vi "Initial Path Plot Sub_VI.vi"(8 "error in (no error)":errorcluster, 10 "Motion Inputs":T3) -> (0 "error out":errorcluster, 1 "Accel Array":dbl[](graph), 2 "Velocity Array":dbl[](graph), 3 "Displacement Array":dbl[](graph), 4 "V max (mm/s)":dbl, 5 "Motion Points":T1, 6 "Dist max (mm)":dbl, 7 "Motion Outputs":T2)   [LabVIEW 2017]
panel:
  out "Waveform Chart":T1(graph)
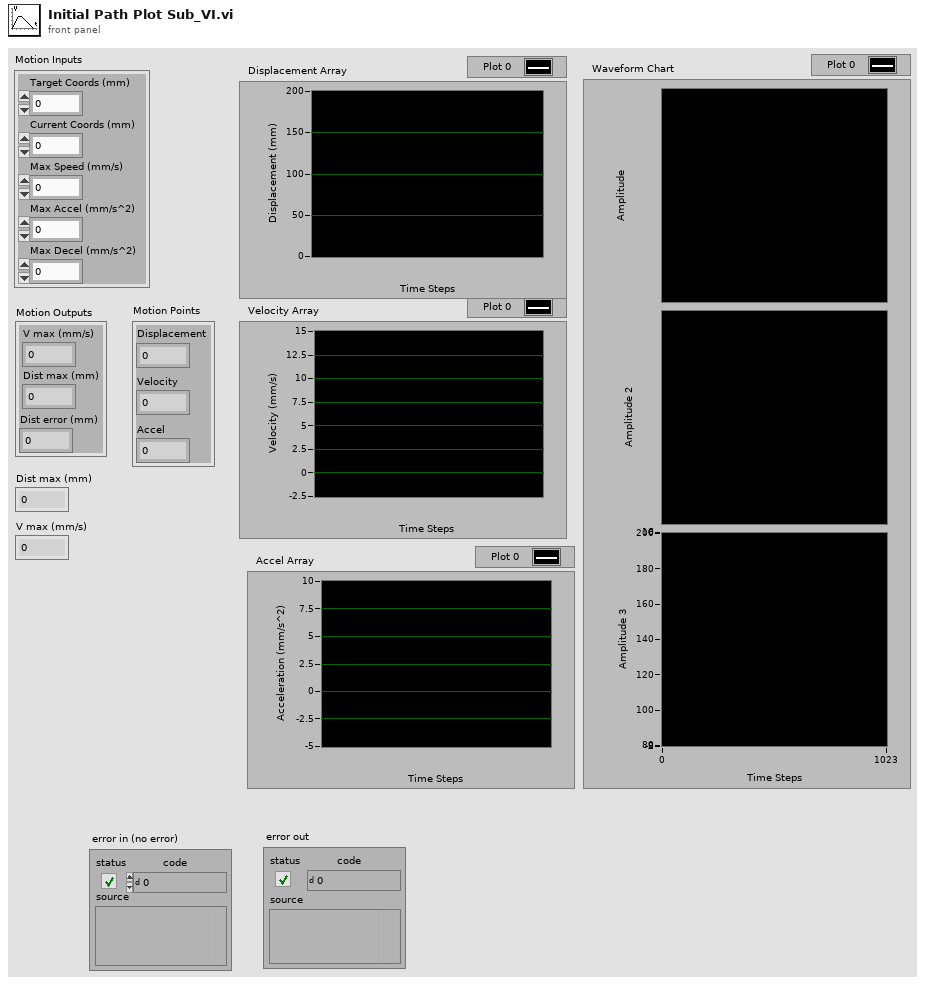
[diagram p1: front panel]
types:
  T1 = cluster{"Accel":dbl, "Velocity":dbl, "Displacement":dbl}
  T2 = cluster{"V max (mm/s)":dbl, "Dist max (mm)":dbl, "Dist error (mm)":dbl}
  T3 = cluster{"Target Coords (mm)":dbl, "Current Coords (mm)":dbl, "Max Speed (mm/s)":dbl, "Max Accel (mm/s^2)":dbl, "Max Decel (mm/s^2)":dbl}
  T4 = cluster{" Distance target (mm)":dbl, "Max Accel (mm/s^2)":dbl, "Max Decel (mm/s^2)":dbl, "Velocity Limit (mm/s) ":dbl, "Time step (s)":dbl}
  T5 = cluster{"Cruising Speed (mm/s)":dbl, "Crusing Time (s)":dbl, "Decel Time (s)":dbl, "Accel Time (s)":dbl, "Total Time (s)":dbl, "Accel Distance (mm)":dbl, "Decel Distance (mm)":dbl, "Crusing Distance (mm)":dbl}
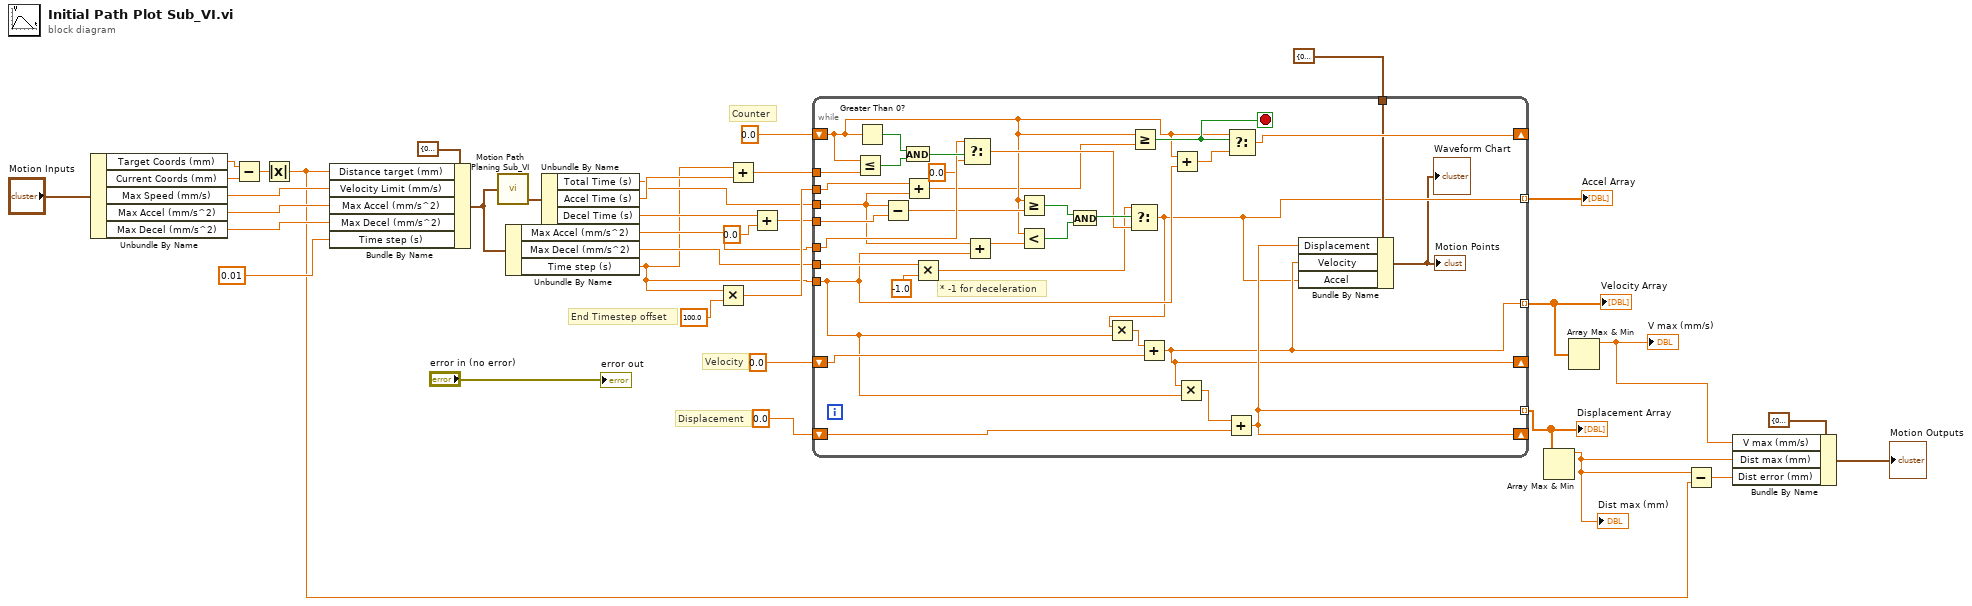
[diagram p0: block diagram]
diagram:
  # "End Timestep offset"
  # "Displacement"
  # "Velocity"
  # "Counter"
  n1 = Unbundle By Name("Motion Inputs") -> ("Target Coords (mm)"=w34:dbl, "Current Coords (mm)"=w35:dbl, "Max Speed (mm/s)"=w32:dbl, "Max Accel (mm/s^2)"=w31:dbl, "Max Decel (mm/s^2)"=w30:dbl)
  n2 = Subtract(x=w34, y=w35) -> (x-y=w21:dbl)
  n3 = Absolute Value(x=w21) -> (abs(x)=w24:dbl)
  n4 = Bundle By Name(cluster=T4 {" Distance target (mm)"=0.0, "Max Accel (mm/s^2)"=0.0, "Max Decel (mm/s^2)"=0.0, "Velocity Limit (mm/s) "=0.0, "Time step (s)"=0.0} ("Motion Planning Inputs"), "Distance target (mm)"=w24, "Velocity Limit (mm/s)"=w32, "Max Accel (mm/s^2)"=w31, "Max Decel (mm/s^2)"=w30, "Time step (s)"=0.01) -> (w28:T4)
  n5 = call "Motion Path Planing Sub_VI.vi"("Motion Planning Inputs"=w28) -> ("Motion Planning Outputs"=w26:T5)  [unwired: 4 in, 2 out]
  n6 = Unbundle By Name(w28) -> ("Max Accel (mm/s^2)"=w3:dbl, "Max Decel (mm/s^2)"=w2:dbl, "Time step (s)"=w1:dbl)
  n7 = Unbundle By Name(w26) -> ("Total Time (s)"=w5:dbl, "Accel Time (s)"=w6:dbl, "Decel Time (s)"=w4:dbl)
  n8 = Multiply(x=w1, y=100.0) -> (x*y=w19:dbl)
  n9 = Add(x=w1, y=w6) -> (x+y=w15:dbl)
  n10 = Add(x=w4, y=0.0) -> (x+y=w16:dbl)
  n11 = while {
    shift-right: [w47] -> _
    shift-left: 0.0 -> [w46]
    tunnel: w15 -> [w69]
    tunnel: w3 -> [w65]
    tunnel: w5 -> [w57]
    tunnel: w16 -> [w62]
    tunnel: [w38] -> w11 mode=indexing
    tunnel: w2 -> [w49]
    shift-right: [w39] -> _
    shift-left: 0.0 -> [w54]
    shift-right: [w41] -> _
    shift-left: 0.0 -> [w52]
    tunnel: [w39] -> w20 mode=indexing
    tunnel: [w41] -> w10 mode=indexing
    tunnel: w1 -> [w44]
    tunnel: w19 -> [w42]
    tunnel: T1 {"Accel"=0.0, "Velocity"=0.0, "Displacement"=0.0} ("Motion Points 2") -> [w40]
    stop <- w55 stop-if-true
    # "* -1 for deceleration"
    n12 = Less Or Equal?(x=w46, y=w69) -> (x <= y?=w67:bool)
    n13 = Greater Than 0?(x=w46) -> (x > 0?=w68:bool)
    n14 = Subtract(x=w57, y=w62) -> (x-y=w63:dbl)
    n15 = And(x=w68, y=w67) -> (x .and. y?=w66:bool)
    n16 = Add(x=w42, y=w57) -> (x+y=w43:dbl)
    n17 = Multiply(x=w49, y=-1.0 ("x")) -> (x*y=w50:dbl)
    n18 = Select(t=w65, s=w66, f=0.0) -> (s? t:f=w58:dbl)
    n19 = Add(x=w57, y=w44) -> (x+y=w45:dbl)
    n20 = Greater Or Equal?(x=w46, y=w63) -> (x >= y?=w61:bool)
    n21 = Less?(x=w46, y=w45) -> (x < y?=w60:bool)
    n22 = And(x=w61, y=w60) -> (x .and. y?=w59:bool)
    n23 = Select(t=w50, s=w59, f=w58) -> (s? t:f=w38:dbl)
    n24 = Multiply(x=w38, y=w44) -> (x*y=w53:dbl)
    n25 = Greater Or Equal?(x=w46, y=w43) -> (x >= y?=w55:bool)
    n26 = Add(x=w53, y=w54) -> (x+y=w39:dbl)
    n27 = Add(x=w46, y=w44) -> (x+y=w56:dbl)
    n28 = Multiply(x=w39, y=w44) -> (x*y=w51:dbl)
    n29 = Add(x=w51, y=w52) -> (x+y=w41:dbl)
    n30 = Select(t=w46, s=w55, f=w56) -> (s? t:f=w47:dbl)
    n31 = Bundle By Name(cluster=w40, "Displacement"=w41, "Velocity"=w39, "Accel"=w38) -> (→"Motion Points" →"Waveform Chart":T1)
  }
  "Accel Array" <- w11
  "Velocity Array" <- w20
  "Displacement Array" <- w10
  n32 = Array Max & Min(array=w10) -> (max value=w8:dbl)  [unwired: 3 out]
  "Dist max (mm)" <- w8
  n33 = Array Max & Min(array=w20) -> (max value=w7:dbl)  [unwired: 3 out]
  "V max (mm/s)" <- w7
  n34 = Subtract(x=w8, y=w24) -> (x-y=w23:dbl)
  n35 = Bundle By Name(cluster=T2 {"V max (mm/s)"=0.0, "Dist max (mm)"=0.0, "Dist error (mm)"=0.0} ("Motion Outputs 2"), "V max (mm/s)"=w7, "Dist max (mm)"=w8, "Dist error (mm)"=w23) -> (→"Motion Outputs":T2)
  "error out" <- "error in (no error)"
